vi "Mux4.vi"(1 "B":bool[](array[boolean])=[FALSE, FALSE, FALSE, FALSE, FALSE, FALSE, FALSE, FALSE, FALSE, FALSE, FALSE, FALSE, FALSE, FALSE, FALSE, FALSE], 2 "A":bool[](array[boolean])=[FALSE, FALSE, FALSE, FALSE, FALSE, FALSE, FALSE, FALSE, FALSE, FALSE, FALSE, FALSE, FALSE, FALSE, FALSE, FALSE], 3 "s0":bool) -> (0 "z":bool[](array[boolean]))   [LabVIEW 2012]
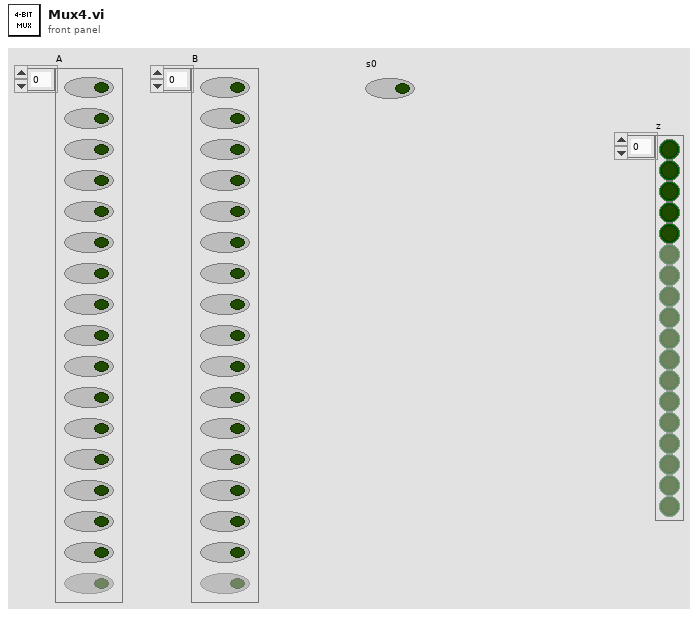
[diagram p1: front panel]
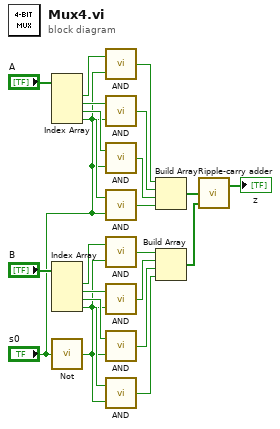
[diagram p0: block diagram]
diagram:
  n1 = Index Array(array="A") -> (element #1=w21:bool, element #2=w20:bool, element #3=w19:bool, element #4=w18:bool)  [unwired: 4 in]
  n2 = Index Array(array="B") -> (element #1=w13:bool, element #2=w12:bool, element #3=w11:bool, element #4=w10:bool)  [unwired: 4 in]
  n3 = call "Not.vi"("In"="s0") -> ("Out"=w8:bool)
  n4 = call "AND.vi"("b"="s0", "a"=w21) -> ("x"=w17:bool)
  n5 = call "AND.vi"("b"="s0", "a"=w20) -> ("x"=w16:bool)
  n6 = call "AND.vi"("b"="s0", "a"=w19) -> ("x"=w15:bool)
  n7 = call "AND.vi"("b"="s0", "a"=w18) -> ("x"=w14:bool)
  n8 = call "AND.vi"("b"=w8, "a"=w13) -> ("x"=w7:bool)
  n9 = call "AND.vi"("b"=w8, "a"=w12) -> ("x"=w6:bool)
  n10 = call "AND.vi"("b"=w8, "a"=w11) -> ("x"=w5:bool)
  n11 = call "AND.vi"("b"=w8, "a"=w10) -> ("x"=w4:bool)
  n12 = Build Array(w17, w16, w15, w14) -> (w3:bool[])
  n13 = Build Array(w7, w6, w5, w4) -> (w2:bool[])
  n14 = call "Ripple-carry adder.vi"("B"=w2, "A"=w3) -> ("S"=→"z":bool[])  [unwired: 1 in, 1 out]
